vi "FTW-Container-Merge.vi"(0 "Container":refnum<class "FTW-Container.lvclass">, 5 "Container to Merge":refnum<class "FTW-Container.lvclass">, 11 "error in":errorcluster) -> (4 "Container out":refnum<class "FTW-Container.lvclass">, 15 "error out":errorcluster)   [LabVIEW 2013, in "FTW-Container.lvclass"]
uses:
  FTW-Container.lvclass
panel:
  # "Inputs"
  # "Outputs"
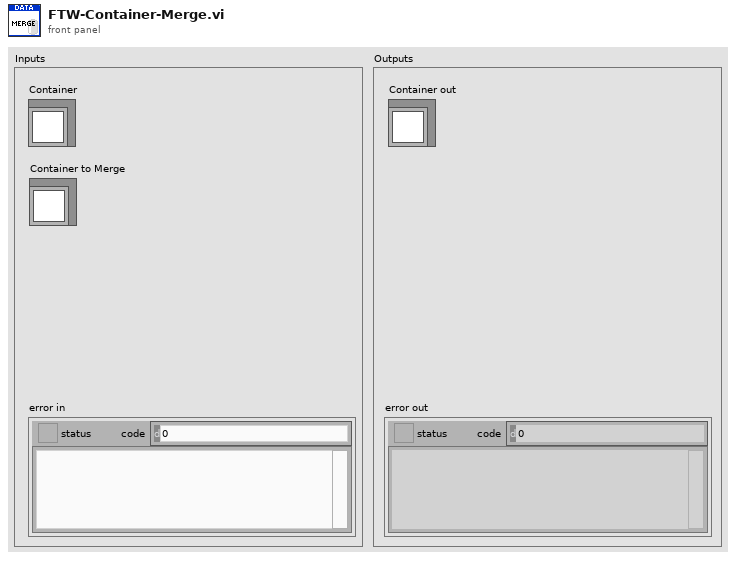
[diagram p1: front panel]
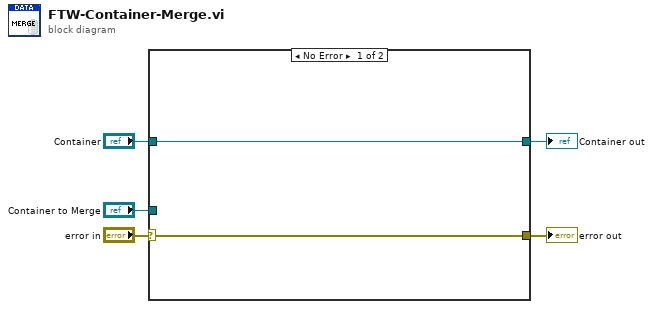
[diagram p0: block diagram]
diagram:
  n1 = case shown="No Error" "error in" {
    selector: "error in" -> [w6 w9]
    tunnel: [w6 w9] -> w5
    tunnel: "Container" -> [w7 w8]
    tunnel: [w7 w8] -> w2
    tunnel: "Container to Merge" -> [_ _]
    frame No Error {
    }
    frame Error {
    }
  }
  "error out" <- w5
  "Container out" <- w2
